vi "Actor Core.vi"(8 "error in":errorcluster, 11 "Nested in":refnum<class "ActorUITemplate.lvclass">) -> (0 "error out":errorcluster, 3 "Actor out":refnum<class "Actor.lvclass">)   [LabVIEW 2021, in "ActorUITemplate.lvclass"]
doc: "(<B>Filename</B>: Actor Framework.lvlib:Actor.lvclass:Actor Core.vi)\n\nReceives messages to the actor, reacts to them, and initiates any error handling that may shut the actor down.\n\nDescendant classes may override this VI to append parallel tasks for the actor to complete while it handles messages. Overrides use the Call Parent Method node."
uses:
  ActorUITemplate.lvclass
  C:/Program Files (x86)/National Instruments/LabVIEW 2021/user.lib/John_Lib/AbstractActorTemplate/AbstractActorTemplate/UIActorTop.lvclass
  C:/Program Files (x86)/National Instruments/LabVIEW 2021/vi.lib/ActorFramework/Actor/Actor.lvclass
  <vilib>/ActorFramework/Actor/Actor.lvclass
  ActorUITemplate.lvclass/ActorUITemplate.ctl
  <vilib>/ActorFramework/Actor/Actor.lvclass/Actor.ctl
  <vilib>/ActorFramework/Message Enqueuer/Message Enqueuer.lvclass/Message Enqueuer.ctl
  <vilib>/ActorFramework/Message Enqueuer/Init from Existing Queue.vi
  <vilib>/ActorFramework/Message Enqueuer/Enqueue.vi
  <vilib>/ActorFramework/Stop Msg/Stop Msg.lvclass
  C:/Program Files (x86)/National Instruments/LabVIEW 2021/vi.lib/ActorFramework/Message/Message.lvclass
  <vilib>/ActorFramework/Message Priority Queue/Priority Enqueue.vi
  <vilib>/ActorFramework/Message Enqueuer/Message Enqueuer.lvclass
  <userlib>/John_Lib/AbstractActorTemplate/AbstractActorTemplate/UIActorTop.lvclass
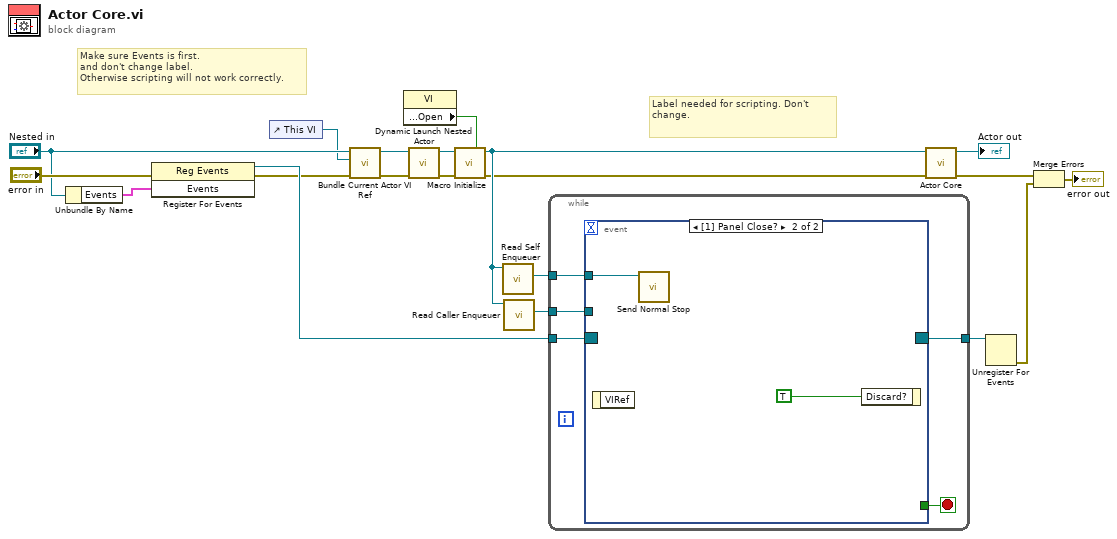
[diagram p0: block diagram]
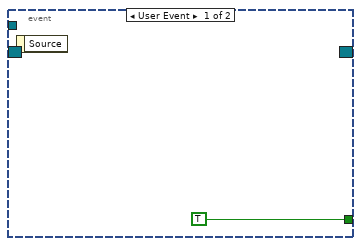
[diagram p2: hidden frame]
diagram:
  # "Label needed for scripting. Don't change."
  # "Make sure Events is first.\nand don't change label.\nOtherwise scripting will not work correctly."
  n1 = Unbundle By Name("Nested in") -> ("Events"=w18:cluster{"Stop":refnum<user-event>})
  n2 = register-events ("Main Register for Events")(error in="error in", w18) -> (reference out=w19:refnum<event-registration>, error out=w3:errorcluster)  [unwired: 1 in]
  n3 = control-ref of="This VI"() -> (w1:refnum<vi>)
  n4 = call <userlib>:"Bundle Current Actor VI Ref.vi"("error in (no error)"=w3, "This VI"=w1, "UI ActorTop in"="Nested in") -> ("error out"=w2:errorcluster, "UI ActorTop out"=w4:refnum<class "ActorUITemplate.lvclass">)  [unwired: 6 in, 1 out]
  n5 = property class="VI"() -> ("Front Panel.Open"=w13:bool)  [unwired: 2 in, 2 out]
  n6 = call-dynamic "Dynamic Launch Nested Actor.vi"("error in (no error)"=w2, "UI ActorTop in"=w4) -> ("error out"=w14:errorcluster, "UI ActorTop out"=w15:refnum<class "ActorUITemplate.lvclass">)  [unwired: 8 in]
  n7 = call-dynamic "Macro Initialize.vi"("Front Panel Window:Open"=w13, "error in (no error)"=w14, "UI ActorTop in"=w15) -> ("error out"=w7:errorcluster, "UI ActorTop out"=w11:refnum<class "ActorUITemplate.lvclass">)  [unwired: 7 in]
  n8 = call <vilib>:"Read Self Enqueuer.vi"("Actor"=w11) -> ("Self Enqueuer"=w16:refnum<class "Message Enqueuer.lvclass">)  [unwired: 10 in]
  n9 = call <vilib>:"Read Caller Enqueuer.vi"("Actor"=w11) -> ("Caller Enqueuer"=w6:refnum<class "Message Enqueuer.lvclass">)  [unwired: 10 in]
  n10 = while {
    tunnel: w19 -> [w25]
    tunnel: [w23] -> w17
    tunnel: w16 -> [w22]
    tunnel: w6 -> [w21]
    stop <- w24 stop-if-true
    n11 = event "UI Events" shown="[1] Panel Close?" {
      selector: w25 -> [_ _]
      dyn-events: [_ _] -> w23
      timeout: _ -> [_ _]
      tunnel: [TRUE _] -> w24
      tunnel: w22 -> [_ w27]
      tunnel: w21 -> [_ _]
      event User Event {
        n12 = event-data() -> ()  [unwired: 1 in, 1 out]
      }
      event Panel Close? {
        n13 = event-data() -> ()  [unwired: 1 in, 1 out]
        n14 = call <vilib>:"Send Normal Stop.vi"("Message Enqueuer"=w27) -> ()  [unwired: 10 in, 1 out]
        n15 = event-data("Discard?"=TRUE) -> ()  [unwired: 1 in, 1 out]
      }
    }
  }
  n16 = call-parent "Actor Core.vi"("error in"=w7, "Actor in"=w11) -> ("error out"=w9:errorcluster, "Actor out"=→"Actor out":refnum<class "Actor.lvclass">)  [unwired: 8 in]
  n17 = Unregister For Events(event registration refnum=w17) -> (error out=w10:errorcluster)  [unwired: 1 in]
  n18 = Merge Errors(w9, w10) -> (→"error out":errorcluster)
